vi "RetrieveMeasurementValues&Attributes.vi"(7 "PlotYScale":u32[](array[numeric]), 8 "error in (no error)":errorcluster, 10 "Variant":variant, 11 "WaveformChartReference":refnum<vi>) -> (0 "error out":errorcluster, 1 "Incorrect DataType?":bool, 2 "Array Of Strings":string[](array[string]), 3 "WaveformArrayOut":waveform(dbl)[](array[waveform]), 4 "LightTower":T1(array[cluster]))   [LabVIEW 2018, in "Visualization.lvlib" / "VisualizeSensor.lvclass"]
doc: "This VI extracts the waveform and string data from the variant data."
uses:
  VisualizeSensor.lvclass
  Sensor/SensorShared/SensorVisulization.ctl
  Sensor/SensorShared/SensorShared.lvlib
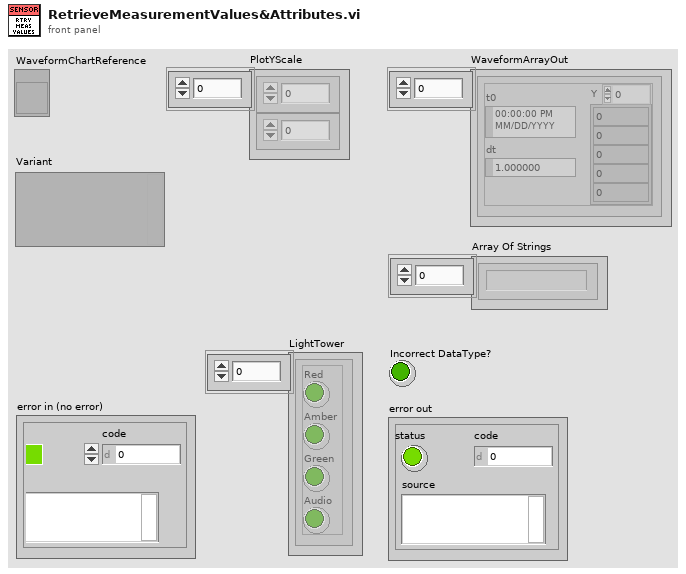
[diagram p1: front panel]
types:
  T1 = cluster{"Red":bool, "Amber":bool, "Green":bool, "Audio":bool}[]
  T2 = typedef "SensorShared.lvlib/SensorVisulization.ctl" = cluster{"Array of Waveforms":waveform(dbl)[], "Array of Strings ":string[], "LightTower":cluster{"Red":bool, "Amber":bool, "Green":bool, "Audio":bool}}
  T3 = cluster{"Red":bool, "Amber":bool, "Green":bool, "Audio":bool}
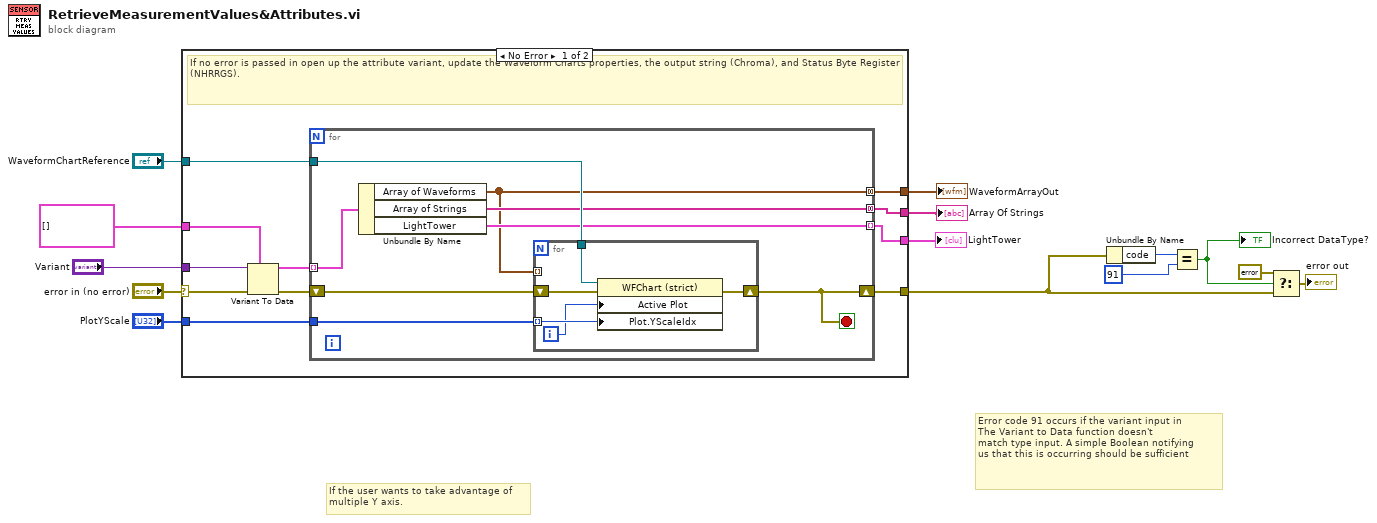
[diagram p0: block diagram]
diagram:
  # "If the user wants to take advantage of \nmultiple Y axis."
  # "Error code 91 occurs if the variant input in \nThe Variant to Data function doesn't \nmatch type input. A simple Boolean notifying \nus that this is occurring should be sufficient"
  n1 = case shown="No Error" "error in (no error)" {
    selector: "error in (no error)" -> [w21 w39]
    tunnel: [w25 w39] -> w6
    tunnel: [w24 _] -> w5
    tunnel: "WaveformChartReference" -> [w22 _]
    tunnel: "PlotYScale" -> [w23 _]
    tunnel: "Variant" -> [w19 _]
    tunnel: T2[] [] -> [w18 _]
    tunnel: [w16 _] -> w3
    tunnel: [w15 _] -> w1
    frame No Error {
      # "If no error is passed in open up the attribute variant, update the Waveform Charts properties, the output string (Chroma), and Status Byte Register (NHRRGS)."
      n2 = Variant To Data(error in=w21, type=w18, Variant=w19) -> (data=w17:T2[], error out=w20:errorcluster)
      n3 = for {
        shift-right: [w31] -> w25
        shift-left: w20 -> [w30]
        tunnel: [w26] -> w24 mode=concatenating
        tunnel: w22 -> [w33]
        tunnel: w23 -> [w32]
        tunnel: w17 -> [w29] mode=indexing
        tunnel: [w28] -> w16 mode=concatenating
        tunnel: [w27] -> w15 mode=indexing
        stop <- w31 stop-if-true
        n4 = Unbundle By Name(w29) -> ("Array of Waveforms"=w26:waveform(dbl)[], "Array of Strings"=w28:string[], "LightTower"=w27:T3)
        n5 = for {
          tunnel: w33 -> [w38]
          tunnel: w32 -> [w37] mode=indexing
          shift-right: [w36] -> w31
          shift-left: w30 -> [w35]
          tunnel: w26 -> [_] mode=indexing
          i -> [w34]
          n6 = property on="Property Node" class="WFChart (strict)"(reference=w38, error in=w35, "Active Plot"=w34, "Plot.YScaleIdx"=w37) -> (error out=w36:errorcluster)  [unwired: 1 out]
        }
      }
    }
    frame Error {
    }
  }
  "WaveformArrayOut" <- w5
  "Array Of Strings" <- w3
  "LightTower" <- w1
  n7 = Unbundle By Name(w6) -> ("code"=w11:i32)
  n8 = Equal?(x=w11, y=91) -> (x = y?=w9:bool)
  "Incorrect DataType?" <- w9
  n9 = Select(t=errorcluster {"status"=FALSE, "code"=0, "source"=""} ("error IO"), s=w9, f=w6) -> (s? t:f=→"error out":errorcluster)
